vi "Write DAQ FIFO.vi"(6 "FIFO Timestamps":T2, 8 "error in (no error)":errorcluster, 9 "Timeout (ms)":i32=100, 10 "Data In":T1[](array[typedef]), 11 "CIF_NIChn_FIFO_DAQ in":refnum<class "CIF_NIChn_FIFO_DAQ.lvclass">) -> (0 "error out":errorcluster, 1 "timed out?":bool, 2 "Data Out":T1[](array[typedef]), 3 "CIF_NIChn_FIFO_DAQ out":refnum<class "CIF_NIChn_FIFO_DAQ.lvclass">)   [LabVIEW 2021, in "CIF_NIChn_FIFO_DAQ.lvclass"]
uses:
  CIF_NIChn_FIFO_DAQ.lvclass
  D:/dev/Packages/Channel_Manager/src/CIFChannels/CIFChannels.lvclass
  D:/dev/Packages/Channel_Manager/src/CIF_NIChn/FIFO_U8/CIF_NIChn_Fifo_U8.lvclass
  ChannelCommon/typedef/TimeStamps.ctl
  ChannelCommon/typedef/Datatype Waveform.ctl
  CIFChannels/CIFChannels.lvclass/CIFChannels.ctl
  CIF_NIChn_FIFO_DAQ.lvclass/CIF_NIChn_FIFO_DAQ.ctl
  FIFO_U8/CIF_NIChn_Fifo_U8.lvclass/CIF_NIChn_Fifo_U8.ctl
  <vilib>/CIF Foundation/CIF Utilities/Statistics/I64/Stats_I64_CIF_U.lvclass/Stats_I64_CIF_U.ctl
  NIChn/CIF_NIChn.lvclass/CIF_NIChn.ctl
  FIFO_U8/Accessors/Read Payload.vi
  NIChn/Accessors/Read CIF Channel.vi
  CIFChannels/Utilities/Update Channel Benchmark.vi
  FIFO_U8/SubVIs/Core Write U8 FIFO.vi/1bad10da-a98b-49ee-b03a-18b497e396df.vi
  FIFO_U8/SubVIs/Core Write U8 FIFO.vi/70f860b1-5d4a-43dc-b0c2-c9446e8447f7.vi
  <vilib>/CIF Foundation/CIF Channels/CIFChannels/Top Level/Write U8 Array.vi
  CIFChannels/Accessors/Read FIFO Header.vi
  ChannelCommon/CIFFIFO/Flatten/DVR Flatten.vi
  FIFO_U8/Accessors/Write Payload.vi
  ChannelCommon/Utilities/Get Waveform DVRs.vi
  CIFChannels/Utilities/Update Flatten Benchmark.vi
  SubVIs/Flatten.vi/587a020d-d764-4ff7-9451-6b801beca2fa.vi
  SubVIs/Flatten.vi/b511efe2-f594-4971-95dc-73ac55586360.vi
  CIFChannels/Accessors/Read FIFO Retry on Timeout.vi
  <vilib>/CIF Foundation/CIF Utilities/Statistics/I64/X1 minus X0.vi
  <vilib>/CIF Foundation/CIF Utilities/Time/System Time/Get System Time.vi
  <vilib>/CIF Foundation/CIF Channels/CIFChannels/SubVIs/Get dll Path.vi
  <vilib>/CIF Foundation/CIF Channels/CIFChannels/SubVIs/Get Requested Size.vi
  <vilib>/CIF Foundation/CIF Utilities/DataTypes/Flatten U64.vi
  CIFChannels/Utilities/Create Flattened FIFO Header.vi
  <vilib>/CIF Foundation/CIF Utilities/Statistics/I64/X1 minus X0.vi/dfabcf33-0dbc-4041-80a5-3dc0c86d2989.vi
  <vilib>/CIF Foundation/CIF Utilities/Time/System Time/LabVIEW Time to TAI Time.vi
  ChannelCommon/Utilities/Flatten Header.vi
  CIFChannels/Utilities/Update FIFO Header.vi
  <vilib>/CIF Foundation/CIF Utilities/Statistics/I64/X1 minus X0.vi/dfabcf33-0dbc-4041-80a5-3dc0c86d2989.vi/9eb60a9a-770f-4d2d-8b3f-8465c267ecc9.vi
  <vilib>/CIF Foundation/CIF Utilities/DataTypes/Flatten I64.vi
  FIFO_U8/CIF_NIChn_Fifo_U8.lvclass
  D:/dev/Packages/Channel_Manager/src/CIF_NIChn/NIChn/CIF_NIChn.lvclass
  D:/dev/Packages/Channel_Manager/src/CIF_NIChn/FIFO_DAQ  not DVR/CIF_NIChn_FIFO_DAQ.lvclass
  ChannelCommon/ChannelCommon.lvlib
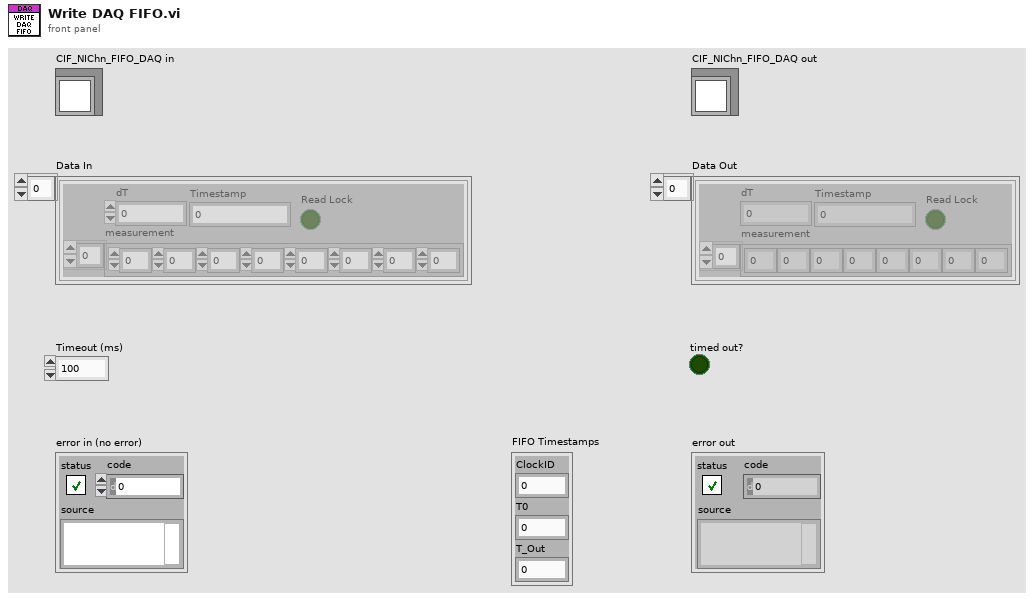
[diagram p1: front panel]
types:
  T1 = typedef "ChannelCommon.lvlib/Datatype Waveform.ctl" = cluster{"measurement":dbl[], "dT":dbl, "Timestamp":i64, "Read Lock":bool}
  T2 = typedef "ChannelCommon.lvlib/TimeStamps.ctl" = cluster{"ClockID":u8, "T0":i64, "T_Out":i64}
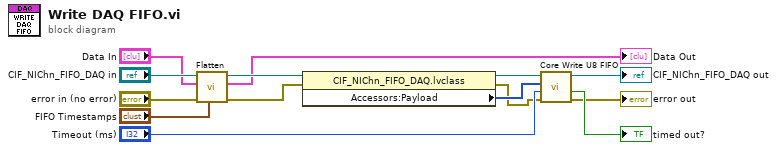
[diagram p0: block diagram]
diagram:
  n1 = call "Flatten.vi"("FIFO Timestamps"="FIFO Timestamps", "error in (no error)"="error in (no error)", "Data In"="Data In", "CIF_NIChn_FIFO_DAQ in"="CIF_NIChn_FIFO_DAQ in") -> ("error out"=w9:errorcluster, "Data Out"=→"Data Out":T1[], "CIF_NIChn_FIFO_DAQ out"=w10:refnum<class "CIF_NIChn_FIFO_DAQ.lvclass">)  [unwired: 5 in]
  n2 = property class="CIF_NIChn_FIFO_DAQ.lvclass"(reference=w10, error in=w9) -> (reference out=w5:refnum<class "CIF_NIChn_FIFO_DAQ.lvclass">, error out=w3:errorcluster, "Accessors:Payload"=w4:u8[])
  n3 = call "Core Write U8 FIFO.vi"("error in (no error)"=w3, "Timeout (ms)"="Timeout (ms)", "U8 With Header"=w4, "CIFFIFO in"=w5) -> ("error out"=→"error out":errorcluster, "timed out?"=→"timed out?":bool, "CIFFIFO out"=→"CIF_NIChn_FIFO_DAQ out":refnum<class "CIF_NIChn_FIFO_DAQ.lvclass">)  [unwired: 5 in]
